vi "sql.vi"() -> ()   [LabVIEW 2016]
uses:
  <vilib>/addons/database/NI_Database_API.lvlib
  ALT irMonitor/Gobal/Global variables.vi
  <vilib>/addons/database/Connection.llb/DB Tools Open Connec (Path).vi
  <vilib>/NI/AMC/AMC.lvlib
  <vilib>/addons/database/Connection.llb/Conn ObjectReference.ctl
  Controles/Objetos.ctl
panel:
  out "error out":errorcluster
  in  "Objetos BBDD":T1
  out "DataBase":bool
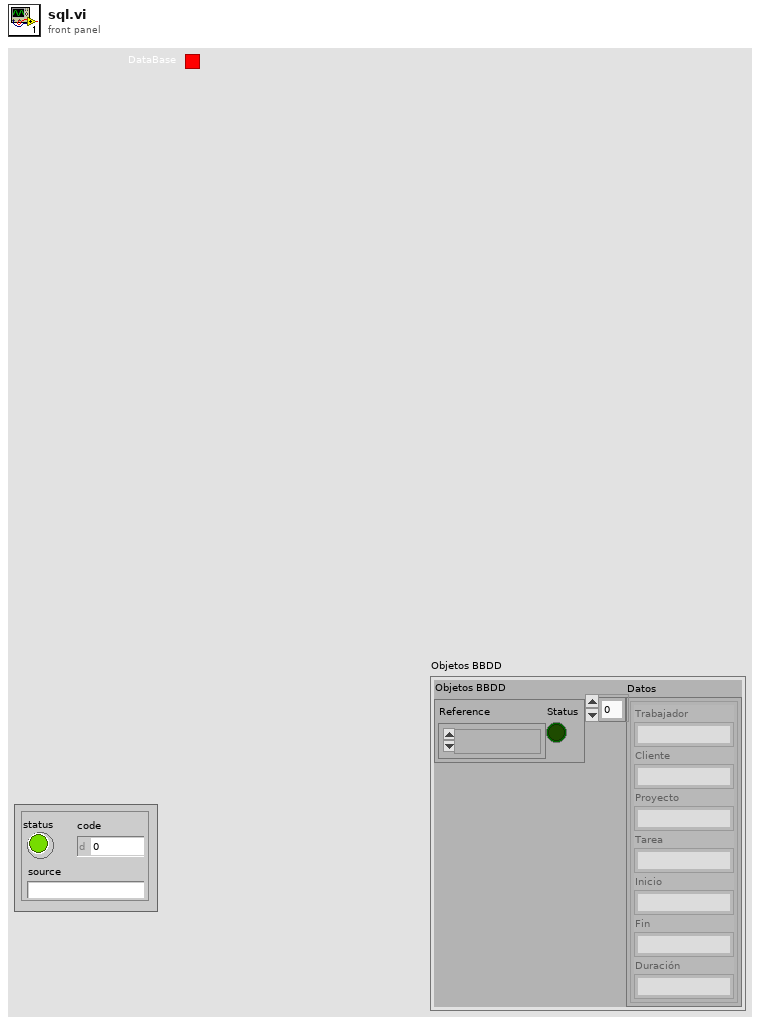
[diagram p1: front panel]
types:
  T1 = typedef "Objetos.ctl" = cluster{"Objetos BBDD":cluster{"Reference":T2, "Status":bool}, "Datos":cluster{"Trabajador":string, "Cliente":string, "Proyecto":string, "Tarea":string, "Inicio":string, "Fin":string, "Duración":string}[]}
  T2 = typedef "NI_Database_API.lvlib/Conn ObjectReference.ctl" = refnum<k1>
  T3 = cluster{"Principal":string, "Base de datos":string, "Dialogs":string, "Log":string, "Cam 1":string, "Cam 2":string, "Cam 3":string, "Cam 4":string, "ioLogik":string}
  T4 = typedef "AMC.lvlib/Message Queue.ctl" = refnum<queue>
  T5 = cluster{"Nombre":void, "Min":void, "Avg":void, "Max":void, "Condición":void, "Resultado":void, "date/time string":string}
  T6 = cluster{"Database UDL":path, "Settings":path, "Ports":path, "Log Events":path}
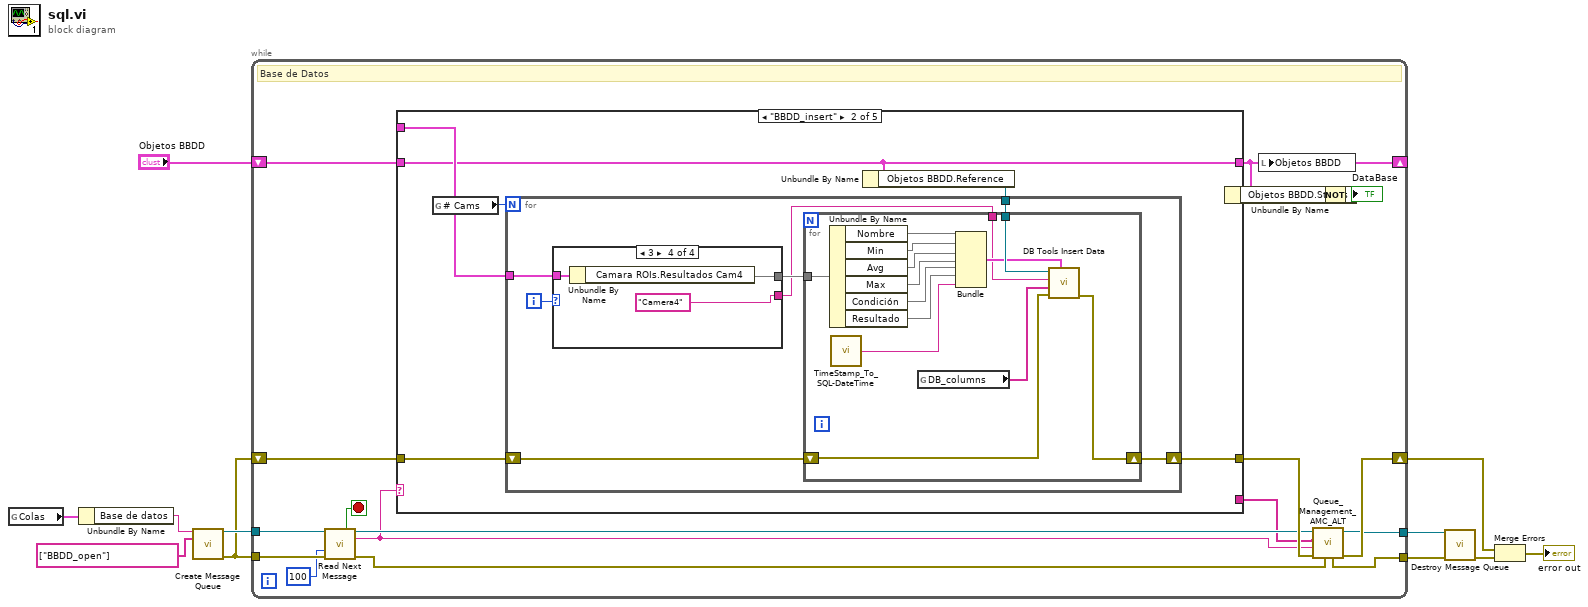
[diagram p0: block diagram]
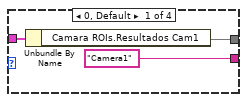
[diagram p3: hidden frame]
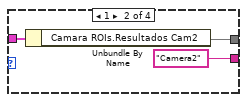
[diagram p4: hidden frame]
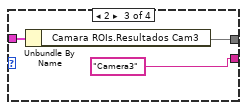
[diagram p5: hidden frame]
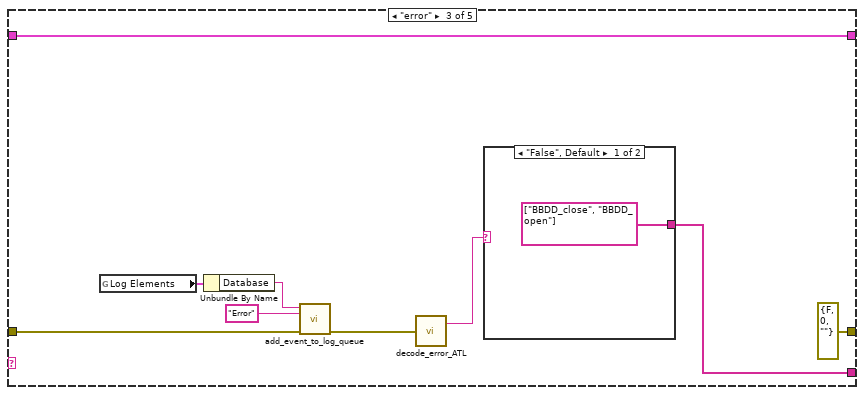
[diagram p6: hidden frame]
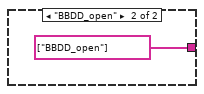
[diagram p7: hidden frame]
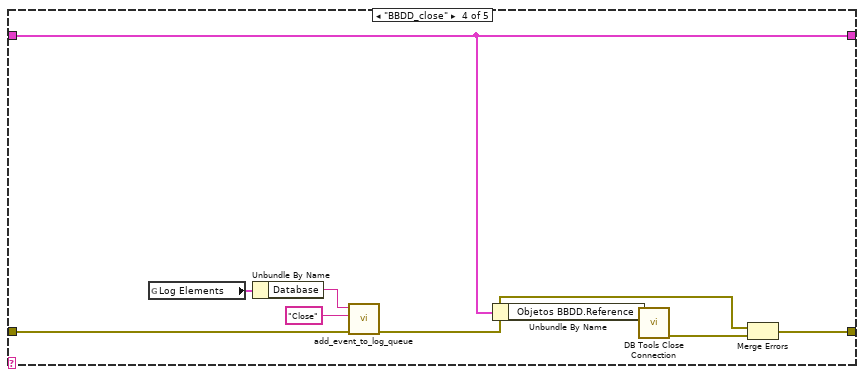
[diagram p8: hidden frame]
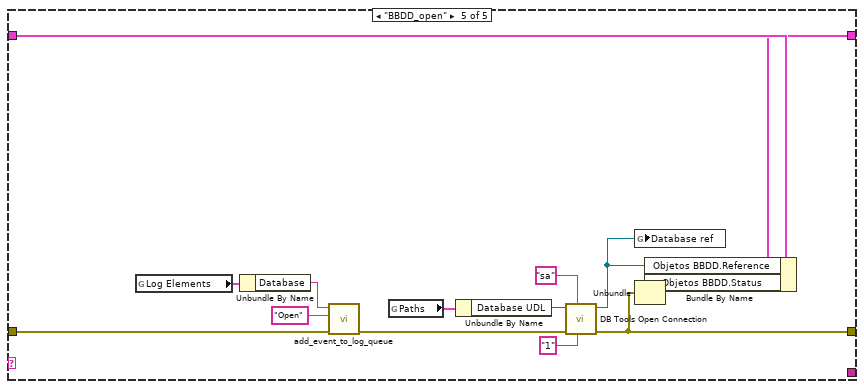
[diagram p9: hidden frame]
diagram:
  n1 = global read "Global variables.vi" "Colas"() -> (w2:T3)
  n2 = Unbundle By Name(w2) -> ("Base de datos"=w1:string)
  n3 = call <vilib>:"Create Message Queue.vi"("message queue name"=w1, "initial message names"=string[] ["BBDD_open"]) -> ("message queue out"=w10:T4, "error out"=w9:errorcluster)  [unwired: 12 in]
  n4 = while {
    tunnel: w10 -> [w28]
    tunnel: w9 -> [w27]
    shift-right: [w15] -> _
    shift-left: "Objetos BBDD" -> [w25]
    shift-right: [w23] -> w4
    shift-left: w9 -> [w26]
    tunnel: [w18] -> w7
    tunnel: [w17] -> w6
    stop <- w12 stop-if-true
    # "Base de Datos"
    n5 = call <vilib>:"Read Next Message.vi"("message queue in"=w28, "timeout (1 ms)"=100, "error in"=w27) -> ("exit process?"=w12:bool, "message queue out"=w21:T4, "message name"=w19:string, "error out"=w20:errorcluster)  [unwired: 5 in, 4 out]
    n6 = case shown="\"BBDD_insert\"" w19 {
      tunnel: w26 -> [w29 w35 w74 w84 w96]
      tunnel: w25 -> [w30 w32 w77 w88 w101]
      tunnel: [w30 w32 w77 w88 w100] -> w15
      tunnel: [w29 w34 errorcluster {"status"=FALSE, "code"=0, "source"=""} ("error out") w86 w97] -> w22
      tunnel: _ -> [_ w33 _ _ _]
      tunnel: [_ _ w75 _ _] -> w16
      frame "Timeout", Default {
      }
      frame "BBDD_insert" {
        n7 = global read "Global variables.vi" "# Cams"() -> (w31:i32)
        n8 = Unbundle By Name(w32) -> ("Objetos BBDD.Reference"=w36:T2)
        n9 = for {
          N: w31 -> [_]
          tunnel: w36 -> [w43]
          shift-right: [w41] -> w34
          shift-left: w35 -> [w42]
          tunnel: w33 -> [w38]
          i -> [w40]
          n10 = case shown="3" w40 {
            tunnel: [w46 w49 w52 w55] -> w39
            tunnel: w38 -> [w45 w48 w51 w54]
            tunnel: ["Camera1" ("table") "Camera2" ("table") "Camera3" ("table") "Camera4" ("table")] -> w37
            frame 0, Default {
              n11 = Unbundle By Name(w45) -> ("Camara ROIs.Resultados Cam1"=w46)
            }
            frame 1 {
              n12 = Unbundle By Name(w48) -> ("Camara ROIs.Resultados Cam2"=w49)
            }
            frame 2 {
              n13 = Unbundle By Name(w51) -> ("Camara ROIs.Resultados Cam3"=w52)
            }
            frame 3 {
              n14 = Unbundle By Name(w54) -> ("Camara ROIs.Resultados Cam4"=w55)
            }
          }
          n15 = for {
            tunnel: w39 -> [w69]
            tunnel: w43 -> [w67]
            shift-right: [w60] -> w41
            shift-left: w42 -> [w61]
            tunnel: w37 -> [w57]
            n16 = Unbundle By Name(w69) -> ("Nombre"=w68, "Min"=w62, "Avg"=w63, "Max"=w64, "Condición"=w65, "Resultado"=w59)
            n17 = call "TimeStamp_To_SQL-DateTime.vi"() -> ("date/time string"=w58:string)  [unwired: 1 in]
            n18 = global read "Global variables.vi" "DB_columns"() -> (w56:string[])
            n19 = Bundle("Nombre"=w68, "Min"=w62, "Avg"=w63, "Max"=w64, "Condición"=w65, "Resultado"=w59, "date/time string"=w58) -> (w66:T5)  [unwired: 1 in]
            n20 = call <vilib>:"DB Tools Insert Data.vi"("data"=w66, "error in (no error)"=w61, "columns"=w56, "table"=w57, "connection reference"=w67) -> ("error out"=w60:errorcluster)  [unwired: 5 in, 1 out]
          }
        }
      }
      frame "error" {
        n21 = global read "Global variables.vi" "Log Elements"() -> (w72:cluster{"Database":string})
        n22 = Unbundle By Name(w72) -> ("Database"=w71:string)
        n23 = call "add_event_to_log_queue.vi"("error in (no error)"=w74, "Evento"="Error", "Elemento"=w71) -> ("error out"=w73:errorcluster)  [unwired: 8 in]
        n24 = call "decode_error_ATL.vi"("error in (no error)"=w73) -> ("case"=w76:string)  [unwired: 1 out]
        n25 = case shown="\"False\", Default" w76 {
          tunnel: [string[] ["BBDD_close", "BBDD_open"] ("message names") string[] ["BBDD_open"] ("message names")] -> w75
          frame "False", Default {
          }
          frame "BBDD_open" {
          }
        }
      }
      frame "BBDD_close" {
        n26 = global read "Global variables.vi" "Log Elements"() -> (w85:cluster{"Database":string})
        n27 = Unbundle By Name(w85) -> ("Database"=w82:string)
        n28 = call "add_event_to_log_queue.vi"("error in (no error)"=w84, "Evento"="Close", "Elemento"=w82) -> ("error out"=w83:errorcluster)  [unwired: 8 in]
        n29 = Unbundle By Name(w88) -> ("Objetos BBDD.Reference"=w89:T2)
        n30 = call <vilib>:"DB Tools Close Connection.vi"("connection reference"=w89) -> ("error out"=w87:errorcluster)  [unwired: 6 in]
        n31 = Merge Errors(w83, w87) -> (w86:errorcluster)
      }
      frame "BBDD_open" {
        n32 = global read "Global variables.vi" "Log Elements"() -> (w94:cluster{"Database":string})
        n33 = Unbundle By Name(w94) -> ("Database"=w91:string)
        n34 = call "add_event_to_log_queue.vi"("error in (no error)"=w96, "Evento"="Open", "Elemento"=w91) -> ("error out"=w95:errorcluster)  [unwired: 8 in]
        n35 = global read "Global variables.vi" "Paths"() -> (w93:T6)
        n36 = Unbundle By Name(w93) -> ("Database UDL"=w92:path)
        n37 = call-poly <vilib>:"DB Tools Open Connection.vi"("password"="1", "userID"="sa", "error in (no error)"=w95, "connection information"=w92) -> ("error out"=w97:errorcluster, "connection reference"=w98:T2)  [unwired: 4 in]
        n38 = global write "Global variables.vi" "Database ref"(w98) -> ()
        n39 = Unbundle(w97) -> ("status"=w99:bool)  [unwired: 2 out]
        n40 = Bundle By Name(cluster=w101, "Objetos BBDD.Reference"=w98, "Objetos BBDD.Status"=w99) -> (w100:T1)
      }
    }
    n41 = Unbundle By Name(w15) -> ("Objetos BBDD.Status"=w14:bool)
    n42 = local write "Objetos BBDD"(w15) -> ()
    n43 = call "Queue_Management_AMC_ALT.vi"("queue error in"=w20, "system error in"=w22, "Case"=w19, "Elementos a cola"=w16, "message queue in"=w21) -> ("system error out"=w23:errorcluster, "message queue out"=w18:T4, "queue error out"=w17:errorcluster)  [unwired: 3 in, 1 out]
    n44 = Not(x=w14) -> (.not. x?=→"DataBase":bool)
  }
  n45 = call <vilib>:"Destroy Message Queue.vi"("message queue in"=w7, "error in"=w6) -> ("error out"=w5:errorcluster)  [unwired: 11 in, 2 out]
  n46 = Merge Errors(w4, w5) -> (→"error out":errorcluster)
